vi "Slice Select.vi"(9 "Count":u8, 11 "Slice":string) -> (1 "Selected":u8, 3 "Cancelled":bool)   [LabVIEW 2019, in "Test Selector.lvlib" / "Test Selector.lvclass"]
uses:
  Test Selector.lvclass
panel:
  in  "Cancel":bool
  in  "Ring":u16(ring)
  in  "OK":bool
  out "String":string
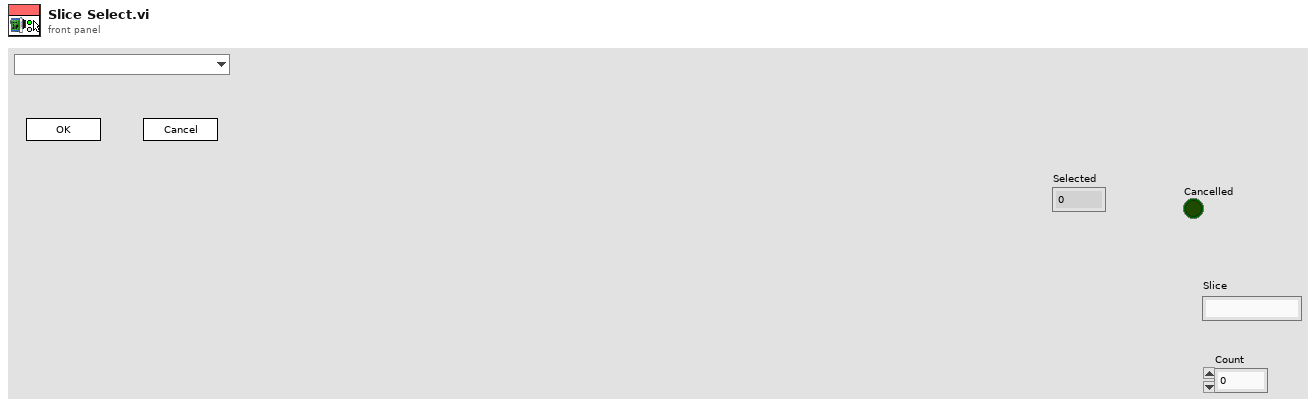
[diagram p1: front panel]
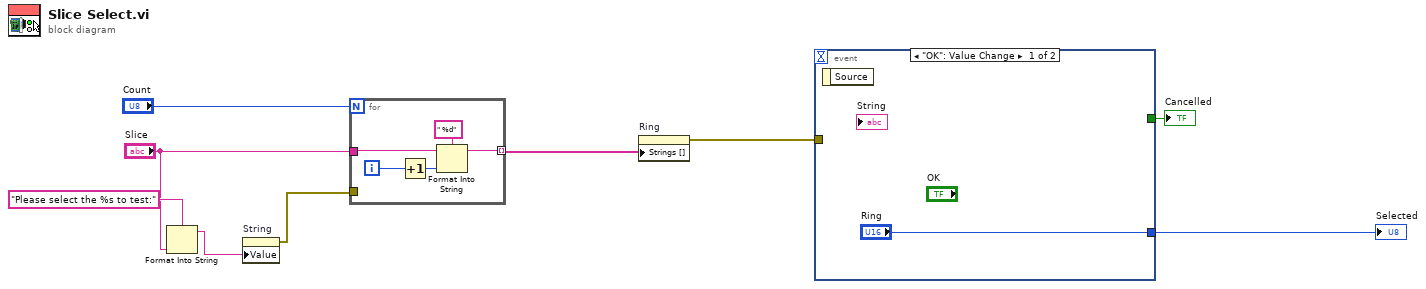
[diagram p0: block diagram]
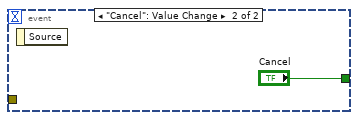
[diagram p2: hidden frame]
diagram:
  n1 = Format Into String(format string="Please select the %s to test:", "Slice") -> (resulting string=w5:string)  [unwired: 2 in, 1 out]
  n2 = property on="String" class="Str"("Value"=w5) -> (error out=w2:errorcluster)  [unwired: 2 in, 1 out]
  n3 = for {
    N: "Count" -> [_]
    tunnel: "Slice" -> [w14]
    tunnel: [w12] -> w9 mode=indexing
    tunnel: w2 -> [_]
    i -> [w10]
    n4 = Increment(x=w10) -> (x+1=w11:i32)
    n5 = Format Into String(format string=" %d", initial string=w14, w11) -> (resulting string=w12:string)  [unwired: 1 in, 1 out]
  }
  n6 = property on="Ring" class="Ring (strict)"("Strings []"=w9) -> (error out=w6:errorcluster)  [unwired: 2 in, 1 out]
  n7 = event shown="[0] \"OK\": Value Change" {
    selector: _ -> [_ _]
    dyn-events: _ -> [_ _]
    timeout: _ -> [_ _]
    tunnel: w6 -> [_ _]
    tunnel: ["Ring" _] -> w7
    tunnel: [_ "Cancel"] -> w8
    event "OK": Value Change {
      n8 = event-data() -> ()  [unwired: 1 in, 1 out]
    }
    event "Cancel": Value Change {
      n9 = event-data() -> ()  [unwired: 1 in, 1 out]
    }
  }
  "Selected" <- w7
  "Cancelled" <- w8
